vi "Read Image Page.vi"(7 "Tiff Bitness":T5(ring), 8 "error in (no error)":errorcluster, 9 "IFDO Info":T4(c390), 10 "Page Info":T2 {"SampleFormat" items=["UINT"=1, "INT"=2, "FP"=3, "VOID"=4, "COMPLEXINT"=5, "COMPLEXFP"=6]; "NewSubFileType" items=["FILETYPE_REDUCEDIMAGE"=1, "FILETYPE_PAGE"=2, "FILETYPE_MASK"=4]; "Compression" items=["COMPRESSION_NONE"=1, "COMPRESSION_CCITTRLE"=2, "COMPRESSION_CCITTFAX3"=3, "COMPRESSION_CCITTFAX4"=4, "COMPRESSION_LZW"=5, "COMPRESSION_OJPEG"=6, "COMPRESSION_JPEG"=7, "COMPRESSION_NEXT"=32766, "COMPRESSION_CCITTRLEW"=32771, "COMPRESSION_PACKBITS"=32773, "COMPRESSION_THUNDERSCAN"=32809, "COMPRESSION_IT8CTPAD"=32895, "COMPRESSION_IT8LW"=32896, "COMPRESSION_IT8MP"=32897, "COMPRESSION_IT8BL"=32898, "COMPRESSION_PIXARFILM"=32908, "COMPRESSION_PIXARLOG"=32909, "COMPRESSION_DEFLATE"=32946, "COMPRESSION_ADOBE_DEFLATE"=8, "COMPRESSION_DSC"=32947, "COMPRESSION_JBIG"=34661, "COMPRESSION_SGILOG"=34676, "COMPRESSION_SGILOG24"=34677, "COMPRESSION_JP2000"=34712]; "PhotometricInterpretation" items=["PHOTOMETRIC_MINISWHITE"=0, "PHOTOMETRIC_MINISBLACK"=1, "PHOTOMETRIC_RGB"=2, "PHOTOMETRIC_PALETTE"=3, "PHOTOMETRIC_MASK"=4, "PHOTOMETRIC_SEPARATED"=5, "PHOTOMETRIC_YCBCR"=6, "PHOTOMETRIC_CIELAB"=8, "PHOTOMETRIC_ICCLAB"=9, "PHOTOMETRIC_ITULAB"=10, "PHOTOMETRIC_LOGL"=32844, "PHOTOMETRIC_LOGLUV"=32845, "CFA"=32803, "LinearRaw"=34892, "DEPTH"=51177]; "ResolutionUnit" items=["RESUNIT_NONE"=1, "RESUNIT_INCH"=2, "RESUNIT_CENTIMETER"=3]}, 11 "Byte Stream File in":refnum<file>) -> (0 "error out":errorcluster, 2 "Details":T1={"ImageDescription"="", "XResolution"=0.0, "YResolution"=0.0, "ResolutionUnit"=enum."Inch", "PhotometricInterpretation"=0, "Compression"=enum."None", "PageName"="", "DocumentName"=""} {"PhotometricInterpretation" items=["PHOTOMETRIC_MINISWHITE"=0, "PHOTOMETRIC_MINISBLACK"=1, "PHOTOMETRIC_RGB"=2, "PHOTOMETRIC_PALETTE"=3, "PHOTOMETRIC_MASK"=4, "PHOTOMETRIC_SEPARATED"=5, "PHOTOMETRIC_YCBCR"=6, "PHOTOMETRIC_CIELAB"=8, "PHOTOMETRIC_ICCLAB"=9, "PHOTOMETRIC_ITULAB"=10, "PHOTOMETRIC_LOGL"=32844, "PHOTOMETRIC_LOGLUV"=32845, "CFA"=32803, "LinearRaw"=34892, "DEPTH"=51177]}, 3 "Variant Strips":variant)   [LabVIEW 2020, in "LV Tiff.lvlib"]
uses:
  LV Tiff.lvlib
  Tiff Data Type.ctl
  Baseline Tags 1.ctl
  Tiff Page Details.ctl
  Tiff Tags.ctl
panel:
  out "Byte Stream File Out":refnum<file>
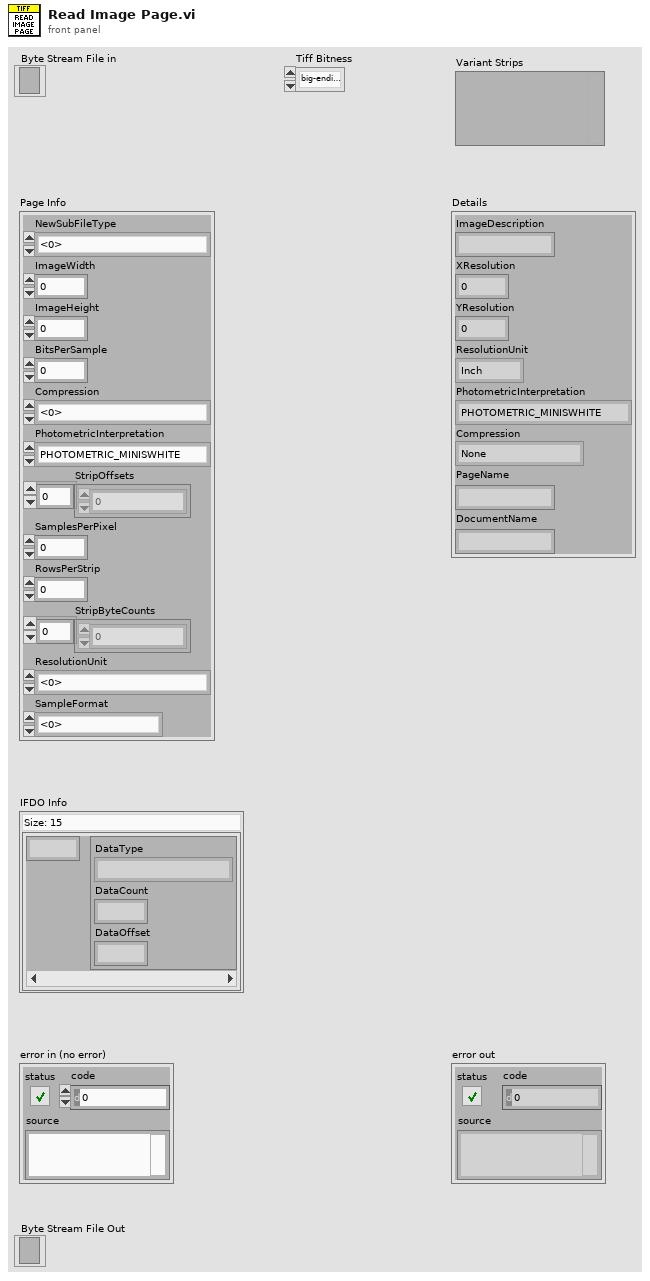
[diagram p1: front panel]
types:
  T1 = typedef "LV Tiff.lvlib/Tiff Page Details.ctl" = cluster{"ImageDescription":string, "XResolution":dbl, "YResolution":dbl, "ResolutionUnit":enum16{"None", "Inch", "Centimeter"}, "PhotometricInterpretation":u16, "Compression":enum16{"None", "Deflate", "JPEG"}, "PageName":string, "DocumentName":string}
  T2 = typedef "LV Tiff.lvlib/Baseline Tags 1.ctl" = cluster{"NewSubFileType":u32, "ImageWidth":u32, "ImageHeight":u32, "BitsPerSample":u16, "Compression":u16, "PhotometricInterpretation":u16, "StripOffsets":u32[], "SamplesPerPixel":u16, "RowsPerStrip":u32, "StripByteCounts":u32[], "ResolutionUnit":u16, "SampleFormat":u16}
  T3 = typedef "LV Tiff.lvlib/Tiff Data Type.ctl" = enum16{"Null", "BYTE", "ASCII", "SHORT", "LONG", "RATIONAL", "SBYTE", "UNDEFINE", "SSHORT", "SLONG", "SRATIONAL", "FLOAT", "DOUBLE"}
  T4 = map{u16, cluster{"DataType":T3, "DataCount":u32, "DataOffset":u32}}
  T5 = enum16{"big-endian, network order", "native, host order", "little-endian"}
  T6 = typedef "LV Tiff.lvlib/Tiff Tags.ctl" = u16
  T7 = typedef "imagedata.ctl" = cluster{"image type":i32, "image depth":i32, "image":u8[], "mask":u8[], "colors":u32[], "Rectangle":cluster{"left":i16, "top":i16, "right":i16, "bottom":i16}}
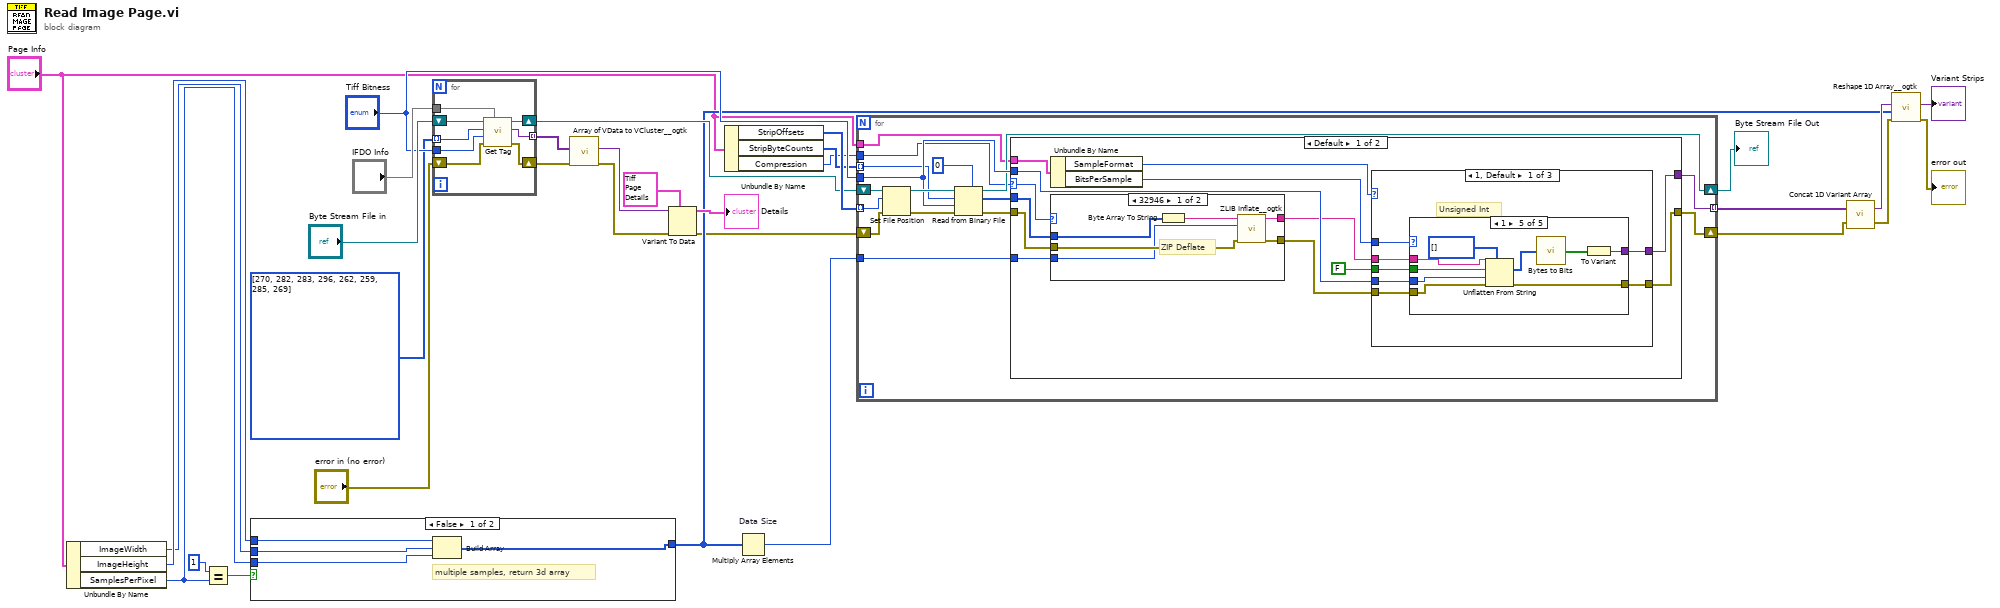
[diagram p0: block diagram]
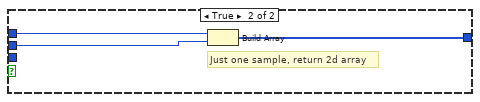
[diagram p2: hidden frame]
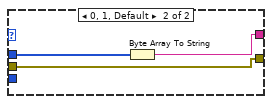
[diagram p3: hidden frame]
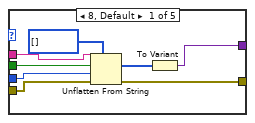
[diagram p4: hidden frame]
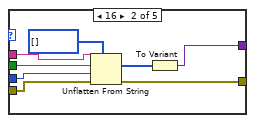
[diagram p5: hidden frame]
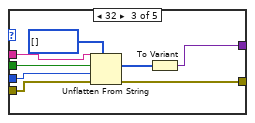
[diagram p6: hidden frame]
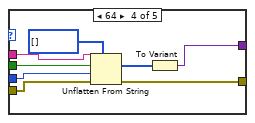
[diagram p7: hidden frame]
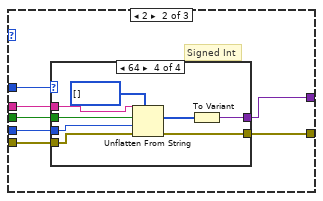
[diagram p8: hidden frame]
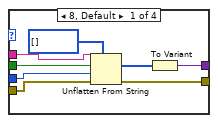
[diagram p9: hidden frame]
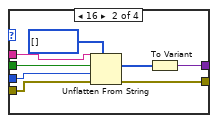
[diagram p10: hidden frame]
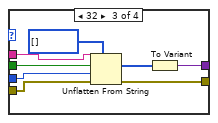
[diagram p11: hidden frame]
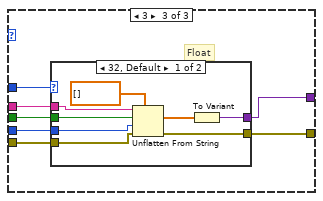
[diagram p12: hidden frame]
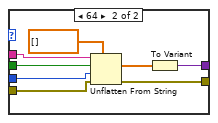
[diagram p13: hidden frame]
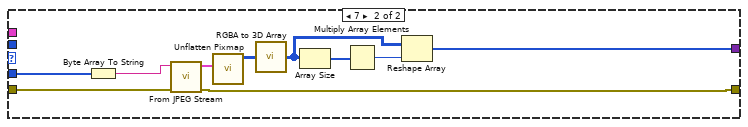
[diagram p14: hidden frame]
diagram:
  w20 = T6[] [270, 282, 283, 296, 262, 259, 285, 269] items=["NewSubFileType"=254, "SubFileType"=255, "ImageWidth"=256, "ImageHeight"=257, "BitsPerSample"=258, "Compression"=259, "PhotometricInterpretation"=262, "Thresholding"=263, "CellWidth"=264, "CellLength"=265, "FillOrder"=266, "DocumentName"=269, "ImageDescription"=270, "Make"=271, "Model"=272, "StripOffsets"=273, "Orientation"=274, "SamplesPerPixel"=277, "RowsPerStrip"=278, "StripByteCounts"=279, "MinSampleValue"=280, "MaxSampleValue"=281, "XResolution"=282, "YResolution"=283, "PlanarConfiguration"=284, "PageName"=285, "XPosition"=286, "YPosition"=287, "FreeOffsets"=288, "FreeByteCounts"=289, "GrayResponseUnit"=290, "GrayResponseCurve"=291, "T4Options[2]"=292, "T6Options[3]"=293, "ResolutionUnit"=296, "PageNumber"=297, "ColorResponseUnit"=300, "TransferFunction[4]"=301, "Software"=305, "DateTime"=306, "Artist"=315, "HostComputer"=316, "Predictor"=317, "WhitePoint"=318, "PrimaryChromaticities"=319, "ColorMap"=320, "HalftoneHints"=321, "TileWidth"=322, "TileLength"=323, "TileOffsets"=324, "TileByteCounts"=325, "BadFaxLines"=326, "CleanFaxData"=327, "ConsecutiveBadFaxLines"=328, "InkSet"=332, "InkNames"=333, "NumberOfInks"=334, "DotRange"=336, "TargetPrinter"=337, "ExtraSamples"=338, "SampleFormat"=339, "SMinSampleValue"=340, "SMaxSampleValue"=341, "TransferRange"=342, "JPEGProc"=512, "JPEGInterchangeFormat"=513, "JPEGInterchangeFormatLength"=514, "JPEGRestartInterval"=515, "JPEGLosslessPredictors"=517, "JPEGPointTransforms"=518, "JPEGQTables"=519, "JPEGDCTTables"=520, "JPEGACTTables"=521, "YCbCrCoefficients"=529, "YCbCrSubSampling"=530, "YCbCrPositioning"=531, "ReferenceBlackWhite"=532, "Copyright"=33432] ("Array")
  n1 = Unbundle By Name("Page Info") -> ("ImageWidth"=w7:u32, "ImageHeight"=w8:u32, "SamplesPerPixel"=w9:u16)
  n2 = Equal?(x=u16 1, y=w9) -> (x = y?=w12:bool)
  n3 = case shown="False" w12 {
    tunnel: w8 -> [w35 w37]
    tunnel: w7 -> [w34 w36]
    tunnel: [w33 w38] -> w11
    tunnel: w9 -> [w32 _]
    frame False {
      # "multiple samples, return 3d array"
      n4 = Build Array(w35, w34, w32) -> (w33:u32[])
    }
    frame True {
      # "Just one sample, return 2d array"
      n5 = Build Array(w37, w36) -> (w38:u32[])
    }
  }
  n6 = for {
    tunnel: [w44] -> w19 mode=indexing
    tunnel: "IFDO Info" -> [w43]
    tunnel: "Tiff Bitness" -> [w41]
    tunnel: w20 -> [w40] mode=indexing
    shift-right: [w45] -> w3
    shift-left: "error in (no error)" -> [w46]
    shift-right: [w39] -> w26
    shift-left: "Byte Stream File in" -> [w42]
    n7 = call "Get Tag.vi"("IFDO"=w43, "error in 2"=w46, "byte order (0:big-endian, network order)"=w41, "Tag ID"=w40, "File Refnum"=w42) -> ("error out"=w45:errorcluster, "Data"=w44:variant, "refnum out"=w39:refnum<file>)  [unwired: 3 in, 1 out]
  }
  n8 = call <userlib>:"Array of VData to VCluster__ogtk.vi"("error in (no error)"=w3, "Array"=w19) -> ("error out"=w5:errorcluster, "VCluster"=w6:variant)  [unwired: 8 in]
  n9 = Variant To Data(error in=w5, type=T1 {"ImageDescription"="", "XResolution"=0.0, "YResolution"=0.0, "ResolutionUnit"=enum."Inch", "PhotometricInterpretation"=0, "Compression"=enum."None", "PageName"="", "DocumentName"=""} ("Details"), Variant=w6) -> (data=→"Details":T1, error out=w2:errorcluster)
  n10 = Unbundle By Name("Page Info") -> ("StripOffsets"=w31:u32[], "StripByteCounts"=w22:u32[], "Compression"=w21:u16)
  n11 = Multiply Array Elements "Data Size"(1:w11) -> (0:w10:u32)
  n12 = for {
    tunnel: w31 -> [w61] mode=indexing
    tunnel: "Tiff Bitness" -> [w54]
    tunnel: [w57] -> w17 mode=indexing
    shift-right: [w59] -> w16
    shift-left: w2 -> [w58]
    shift-right: [w53] -> w24
    shift-left: w26 -> [w62]
    tunnel: w22 -> [w52] mode=indexing
    tunnel: w21 -> [w51]
    tunnel: w10 -> [w48]
    tunnel: "Page Info" -> [w47]
    n13 = Set File Position(offset (in bytes) (0)=w61, refnum=w62, error in=w58) -> (refnum out=w56:refnum<file>, error out=w60:errorcluster)  [unwired: 1 in]
    n14 = Read from Binary File(5:u8 0, 8:w60, 9:w54, 10:w52, 11:w56) -> (0:w49:errorcluster, 2:w50:u8[], 3:w53:refnum<file>)  [unwired: 1 in, 1 out]
    n15 = case shown="Default" w51 {
      selector: w51 -> [w71 _]
      tunnel: [w75 w200] -> w59
      tunnel: [w74 w199] -> w57
      tunnel: w54 -> [w73 _]
      tunnel: w50 -> [w70 w204]
      tunnel: w49 -> [w68 w203]
      tunnel: w48 -> [w66 _]
      tunnel: w47 -> [w65 _]
      frame Default {
        n16 = Unbundle By Name(w65) -> ("SampleFormat"=w64:u16, "BitsPerSample"=w63:u16)
        n17 = case shown="32946" w71 {
          tunnel: w70 -> [w81 w84]
          tunnel: [w79 w83] -> w69
          tunnel: w68 -> [w78 w82]
          tunnel: [w77 w82] -> w67
          tunnel: w66 -> [w76 _]
          frame 32946 {
            # "ZIP Deflate"
            n18 = Byte Array To String(unsigned byte array=w81) -> (string=w80:string)
            n19 = call <userlib>:"ZLIB Inflate__ogtk.vi"("error in (no error)"=w78, "expected length (try out)"=w76, "input"=w80) -> ("error out"=w77:errorcluster, "inflated output"=w79:string)  [unwired: 2 in, 1 out]
          }
          frame 0, 1, Default {
            n20 = Byte Array To String(unsigned byte array=w84) -> (string=w83:string)
          }
        }
        n21 = case shown="1, Default" w64 {
          tunnel: w69 -> [w91 w139 w178]
          tunnel: w73 -> [w90 w138 w177]
          tunnel: FALSE -> [w89 w137 w176]
          tunnel: [w88 w136 w175] -> w74
          tunnel: w67 -> [w87 w135 w174]
          tunnel: w63 -> [w86 w134 w173]
          tunnel: [w85 w133 w172] -> w75
          frame 1, Default {
            # "Unsigned Int"
            n22 = case shown="1" w86 {
              tunnel: w91 -> [w93 w107 w115 w123 w132]
              tunnel: w90 -> [w99 w106 w114 w122 w131]
              tunnel: w89 -> [w92 w105 w113 w121 w130]
              tunnel: [w98 w104 w112 w120 w129] -> w88
              tunnel: w87 -> [w97 w103 w111 w119 w128]
              tunnel: [w95 w101 w109 w117 w126] -> w85
              frame 8, Default {
                n23 = Unflatten From String(type=u8[] [], binary string=w93, data includes array or string size? (T)=w92, byte order (0:big-endian, network order)=w99, error in (no error)=w97) -> (value=w94:u8[], error out=w95:errorcluster)  [unwired: 1 out]
                n24 = To Variant(anything=w94) -> (Variant=w98:variant)
              }
              frame 16 {
                n25 = Unflatten From String(type=u16[] [], binary string=w107, data includes array or string size? (T)=w105, byte order (0:big-endian, network order)=w106, error in (no error)=w103) -> (value=w100:u16[], error out=w101:errorcluster)  [unwired: 1 out]
                n26 = To Variant(anything=w100) -> (Variant=w104:variant)
              }
              frame 32 {
                n27 = Unflatten From String(type=u32[] [], binary string=w115, data includes array or string size? (T)=w113, byte order (0:big-endian, network order)=w114, error in (no error)=w111) -> (value=w108:u32[], error out=w109:errorcluster)  [unwired: 1 out]
                n28 = To Variant(anything=w108) -> (Variant=w112:variant)
              }
              frame 64 {
                n29 = Unflatten From String(type=u64[] [], binary string=w123, data includes array or string size? (T)=w121, byte order (0:big-endian, network order)=w122, error in (no error)=w119) -> (value=w116:u64[], error out=w117:errorcluster)  [unwired: 1 out]
                n30 = To Variant(anything=w116) -> (Variant=w120:variant)
              }
              frame 1 {
                n31 = Unflatten From String(type=u8[] [], binary string=w132, data includes array or string size? (T)=w130, byte order (0:big-endian, network order)=w131, error in (no error)=w128) -> (value=w125:u8[], error out=w126:errorcluster)  [unwired: 1 out]
                n32 = call "Bytes to Bits.vi"("Bytes"=w125) -> ("Bits"=w124:bool[])
                n33 = To Variant(anything=w124) -> (Variant=w129:variant)
              }
            }
          }
          frame 2 {
            # "Signed Int"
            n34 = case shown="64" w134 {
              tunnel: w139 -> [w147 w155 w163 w171]
              tunnel: w138 -> [w146 w154 w162 w170]
              tunnel: w137 -> [w145 w153 w161 w169]
              tunnel: [w144 w152 w160 w168] -> w136
              tunnel: w135 -> [w143 w151 w159 w167]
              tunnel: [w141 w149 w157 w165] -> w133
              frame 8, Default {
                n35 = Unflatten From String(type=i8[] [], binary string=w147, data includes array or string size? (T)=w145, byte order (0:big-endian, network order)=w146, error in (no error)=w143) -> (value=w140:i8[], error out=w141:errorcluster)  [unwired: 1 out]
                n36 = To Variant(anything=w140) -> (Variant=w144:variant)
              }
              frame 16 {
                n37 = Unflatten From String(type=i16[] [], binary string=w155, data includes array or string size? (T)=w153, byte order (0:big-endian, network order)=w154, error in (no error)=w151) -> (value=w148:i16[], error out=w149:errorcluster)  [unwired: 1 out]
                n38 = To Variant(anything=w148) -> (Variant=w152:variant)
              }
              frame 32 {
                n39 = Unflatten From String(type=i32[] [], binary string=w163, data includes array or string size? (T)=w161, byte order (0:big-endian, network order)=w162, error in (no error)=w159) -> (value=w156:i32[], error out=w157:errorcluster)  [unwired: 1 out]
                n40 = To Variant(anything=w156) -> (Variant=w160:variant)
              }
              frame 64 {
                n41 = Unflatten From String(type=i64[] [], binary string=w171, data includes array or string size? (T)=w169, byte order (0:big-endian, network order)=w170, error in (no error)=w167) -> (value=w164:i64[], error out=w165:errorcluster)  [unwired: 1 out]
                n42 = To Variant(anything=w164) -> (Variant=w168:variant)
              }
            }
          }
          frame 3 {
            # "Float"
            n43 = case shown="32, Default" w173 {
              tunnel: w178 -> [w186 w194]
              tunnel: w177 -> [w185 w193]
              tunnel: w176 -> [w184 w192]
              tunnel: [w183 w191] -> w175
              tunnel: w174 -> [w182 w190]
              tunnel: [w180 w188] -> w172
              frame 32, Default {
                n44 = Unflatten From String(type=sgl[] [], binary string=w186, data includes array or string size? (T)=w184, byte order (0:big-endian, network order)=w185, error in (no error)=w182) -> (value=w179:sgl[], error out=w180:errorcluster)  [unwired: 1 out]
                n45 = To Variant(anything=w179) -> (Variant=w183:variant)
              }
              frame 64 {
                n46 = Unflatten From String(type=dbl[] [], binary string=w194, data includes array or string size? (T)=w192, byte order (0:big-endian, network order)=w193, error in (no error)=w190) -> (value=w187:dbl[], error out=w188:errorcluster)  [unwired: 1 out]
                n47 = To Variant(anything=w187) -> (Variant=w191:variant)
              }
            }
          }
        }
      }
      frame 7 {
        n48 = Byte Array To String(unsigned byte array=w204) -> (string=w202:string)
        n49 = call "From JPEG Stream.vi"("error in (no error)"=w203, "Byte Stream"=w202) -> ("error out"=w200:errorcluster, "image data"=w201:T7)  [unwired: 8 in]
        n50 = call <vilib>:"Unflatten Pixmap.vi"("image data"=w201) -> ("24-bit pixmap"=w196:u32[][])  [unwired: 4 in, 6 out]
        n51 = call "RGBA to 3D Array.vi"("24-bit pixmap"=w196) -> ("RGB Array"=w195:u8[][][])  [unwired: 1 in]
        n52 = Array Size(array=w195) -> (size(s)=w198:i32[])
        n53 = Multiply Array Elements(1:w198) -> (0:w197:i32)
        n54 = Reshape Array(w195, w197) -> (w199:u8[])
      }
    }
  }
  "Byte Stream File Out" <- w24
  n55 = call "Concat 1D Variant Array.vi"("error in (no error)"=w16, "Array"=w17) -> ("error out"=w15:errorcluster, "Variant"=w14:variant)
  n56 = call <userlib>:"Reshape 1D Array__ogtk.vi"("error in (no error)"=w15, "Size(s)"=w11, "1D Array"=w14) -> ("error out"=→"error out":errorcluster, "Reshaped VArray"=→"Variant Strips":variant)  [unwired: 7 in]
